vi "Get UI Control Value.vi"(8 "error in (no error)":errorcluster, 10 "VI Ref":refnum<vi>, 11 "Double Parameter in":refnum<class "Double Parameter.lvclass">) -> (0 "error out":errorcluster, 3 "Double Parameter out":refnum<class "Double Parameter.lvclass">)   [LabVIEW 2019, in "CD Parameter Manager API.lvlib" / "Double Parameter.lvclass"]
uses:
  Double Parameter.lvclass
  Double Parameter.lvclass/Double Parameter.ctl
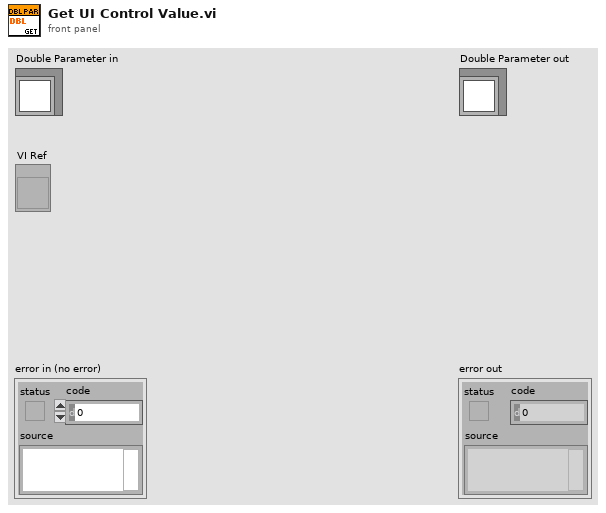
[diagram p1: front panel]
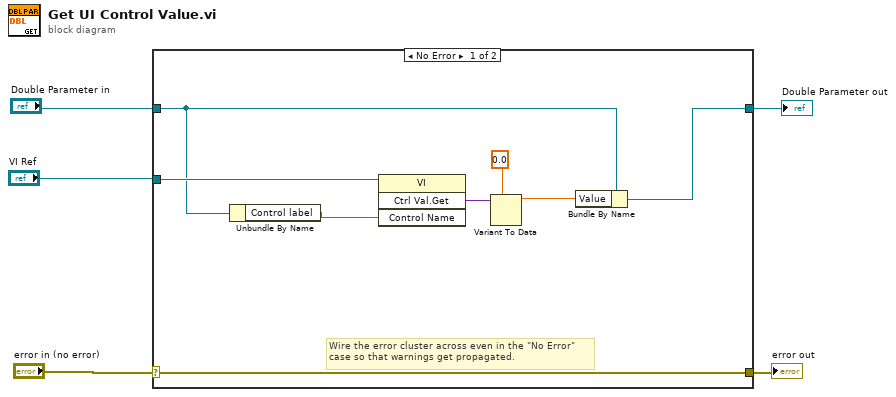
[diagram p0: block diagram]
diagram:
  n1 = case shown="No Error" "error in (no error)" {
    selector: "error in (no error)" -> [w13 w15]
    tunnel: [w13 w15] -> w5
    tunnel: [w9 w14] -> w4
    tunnel: "Double Parameter in" -> [w10 w14]
    tunnel: "VI Ref" -> [w11 _]
    frame No Error {
      # "Wire the error cluster across even in the \"No Error\"\ncase so that warnings get propagated."
      n2 = Unbundle By Name(w10) -> ("Control label"=w12:string)
      n3 = invoke class="VI" method="Ctrl Val.Get"(reference=w11, "Control Name"=w12) -> ("Get Control Value Variant"=w8:variant)  [unwired: 2 in, 3 out]
      n4 = Variant To Data(type=0.0 ("Value"), Variant=w8) -> (data=w7:dbl)  [unwired: 1 in, 1 out]
      n5 = Bundle By Name(cluster=w10, "Value"=w7) -> (w9:refnum<class "Double Parameter.lvclass">)
    }
    frame Error {
    }
  }
  "error out" <- w5
  "Double Parameter out" <- w4
